vi "EmerBeta.vi"(1 "array in":dbl[](array[numeric]), 2 "IR Sensors":dbl[](array[numeric])) -> (0 "appended array":dbl[](array[numeric]))   [LabVIEW 2019]
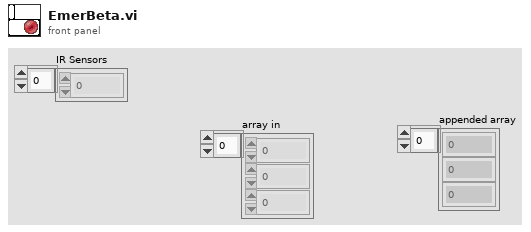
[diagram p1: front panel]
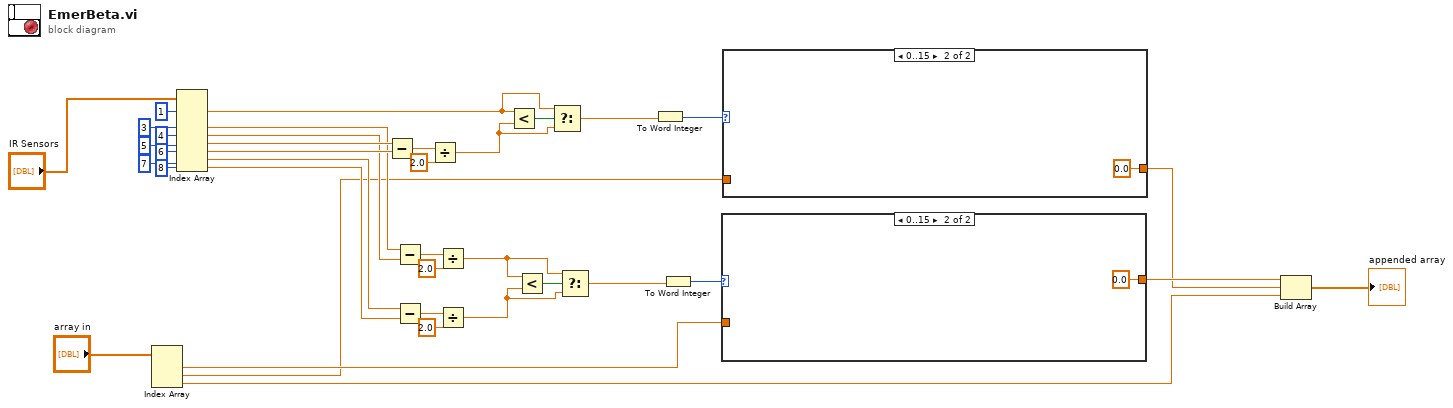
[diagram p0: block diagram]
diagram:
  n1 = Index Array(array="array in") -> (element #1=w6:dbl, element #2=w5:dbl, element #3=w1:dbl)  [unwired: 3 in]
  n2 = Index Array(array="IR Sensors", index #1=1 ("index"), index #3=3 ("index"), index #4=4 ("index"), index #5=5 ("index"), index #6=6 ("index"), index #7=7 ("index"), index #8=8 ("index")) -> (element #1=w28:dbl, element #3=w10:dbl, element #4=w9:dbl, element #5=w26:dbl, element #6=w27:dbl, element #7=w8:dbl, element #8=w7:dbl)  [unwired: 1 in, 1 out]
  n3 = Subtract(x=w26, y=w27) -> (x-y=w25:dbl)
  n4 = Subtract(x=w10, y=w9) -> (x-y=w12:dbl)
  n5 = Subtract(x=w8, y=w7) -> (x-y=w16:dbl)
  n6 = Divide(x=w25, y=2.0) -> (x/y=w23:dbl)
  n7 = Divide(x=w12, y=2.0) -> (x/y=w11:dbl)
  n8 = Divide(x=w16, y=2.0) -> (x/y=w18:dbl)
  n9 = Less?(x=w28, y=w23) -> (x < y?=w35:bool)
  n10 = Less?(x=w11, y=w18) -> (x < y?=w15:bool)
  n11 = Select(t=w28, s=w35, f=w23) -> (s? t:f=w20:dbl)
  n12 = Select(t=w11, s=w15, f=w18) -> (s? t:f=w19:dbl)
  n13 = To Word Integer(number=w20) -> (16bit integer=w21:i16)
  n14 = To Word Integer(number=w19) -> (16bit integer=w14:i16)
  n15 = case shown="0..15" w14 {
    tunnel: w6 -> [w38 _]
    tunnel: [w38 0.0 ("element")] -> w3
    frame Default {
    }
    frame 0..15 {
    }
  }
  n16 = case shown="0..15" w21 {
    tunnel: w5 -> [w40 _]
    tunnel: [w40 0.0 ("element")] -> w2
    frame Default {
    }
    frame 0..15 {
    }
  }
  n17 = Build Array(w3, w2, w1) -> (→"appended array":dbl[])
